vi "Script-Window.vi"(7 "Name(\"\" to use uuid)":string="CSM-Script-Window") -> ()   [LabVIEW 2017, in "DebugConsole.lvlib"]
uses:
  DebugConsole.lvlib
  _BroadcastDef.ctl
  3367f4d9-0615-441f-a9d9-7b84bb446da0.vi
  bf08bd7f-6dab-4e10-8f7c-f5bade8a8a48.vi
  AdvanceAPI/CSM - Revert Arguments-Safe String.vi
  AdvanceAPI/CSM - Keywords.vi
  _csmlite/_PassAllowedMessage - Mapping.vi
  _Shared/Trim Single-line Text.vi
  _Polymophic/Build Synchronous Message with Arguments.vi
  _Polymophic/Build Asynchronous Message with Arguments.vi
  <vilib>/Utility/Data Type/Get Type Information.vi
  _csmHelper/lvcsmFile/lvcsm File Path.vi
  <vilib>/Utility/config.llb/Open Config Data.vi
  <vilib>/Utility/config.llb/Read Key.vi
  <vilib>/Utility/config.llb/Read Key (Boolean).vi
  <vilib>/Utility/config.llb/Read Key (String).vi
  <vilib>/Utility/Data Type/Get Array Information.vi
  <vilib>/Utility/config.llb/Get Key Names.vi
  _csmHelper/lvcsmFile/Path to lvcsm String.vi
  _csmHelper/lvcsmFile/lvcsm String to Path.vi
  <vilib>/Utility/config.llb/Read Key (I32).vi
  <vilib>/Utility/config.llb/Read Key (Double).vi
  <vilib>/Utility/config.llb/Close Config Data.vi
  _csmHelper/lvcsmFile/_Array of VData to VCluster.vi
  <vilib>/Utility/config.llb/Write Key.vi
  <vilib>/Utility/config.llb/Write Key (Boolean).vi
  <vilib>/Utility/config.llb/Remove Key.vi
  <vilib>/Utility/config.llb/Write Key (String).vi
  <vilib>/Utility/config.llb/Write Key (I32).vi
  <vilib>/Utility/config.llb/Write Key (Double).vi
  Communicable State Machine.lvlib
  _csmlite/_csmlite.lvlib
  _csmHelper/lvcsmFile/lvcsm File Support.lvlib
  _Shared/CSM Shared.lvlib
panel:
  in  "List":string(combo)
  in  "Delete":bool
  in  "Save":bool
  out "Running":bool
  in  "Stop":bool
  in  "Play":bool
  in  "Refresh":bool
  in  "Scripts":i32(listbox)
  out "statusbar":string
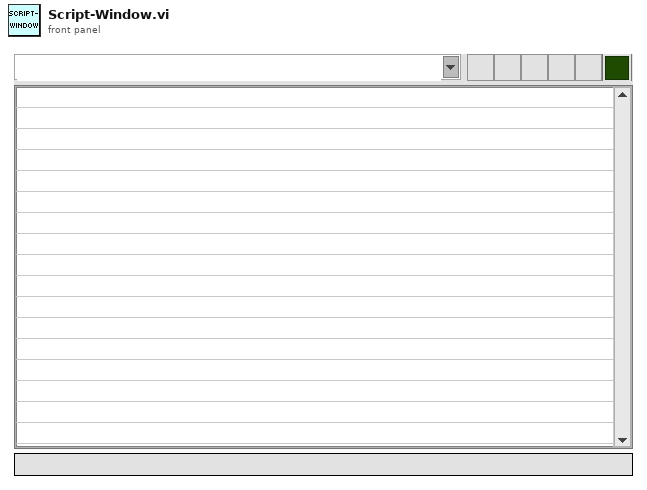
[diagram p1: front panel]
types:
  T1 = enum32{"Invalid", "Standard", "Closed", "Hidden", "Minimized", "Maximized"}
  T2 = enum32{"invalid app kind", "Development System", "Run Time System", "Student Edition", "Embedded LabVIEW", "Evaluation", "Custom"}
  T3 = typedef "DebugConsole.lvlib/_BroadcastDef.ctl" = enum16{"<no action>", "Macro: Exit", "CSM: Module List Changed", "CSM: Scripts Changed", "CSM: Registration Changed", "CSM: Module Selected", "CSM: Message Excuted", "CSM: Broadcast Excuted", "CSM: Registration Action Excuted"}
  T4 = typedef "LVPoint32TypeDef.ctl" = cluster{"Horizontal":i32, "Vertical":i32}
  T5 = cluster{"Current VI Reference":refnum<vi>, "Close Panel on Exit?":bool}
  T6 = cluster{"Core":cluster{"Current VI Reference":refnum<vi>, "Close Panel on Exit?":bool}, "CSMScripts":cluster{"Value":string, "Scripts":cluster{"Target":string, "Function":string, "Parameters":string, "Async Call?":bool}[]}[]}
  T7 = cluster{"Value":string, "Scripts":cluster{"Target":string, "Function":string, "Parameters":string, "Async Call?":bool}[]}[]
  T8 = cluster{"Value":string, "Scripts":cluster{"Target":string, "Function":string, "Parameters":string, "Async Call?":bool}[]}
  T9 = cluster{"Target":string, "Function":string, "Parameters":string, "Async Call?":bool}[]
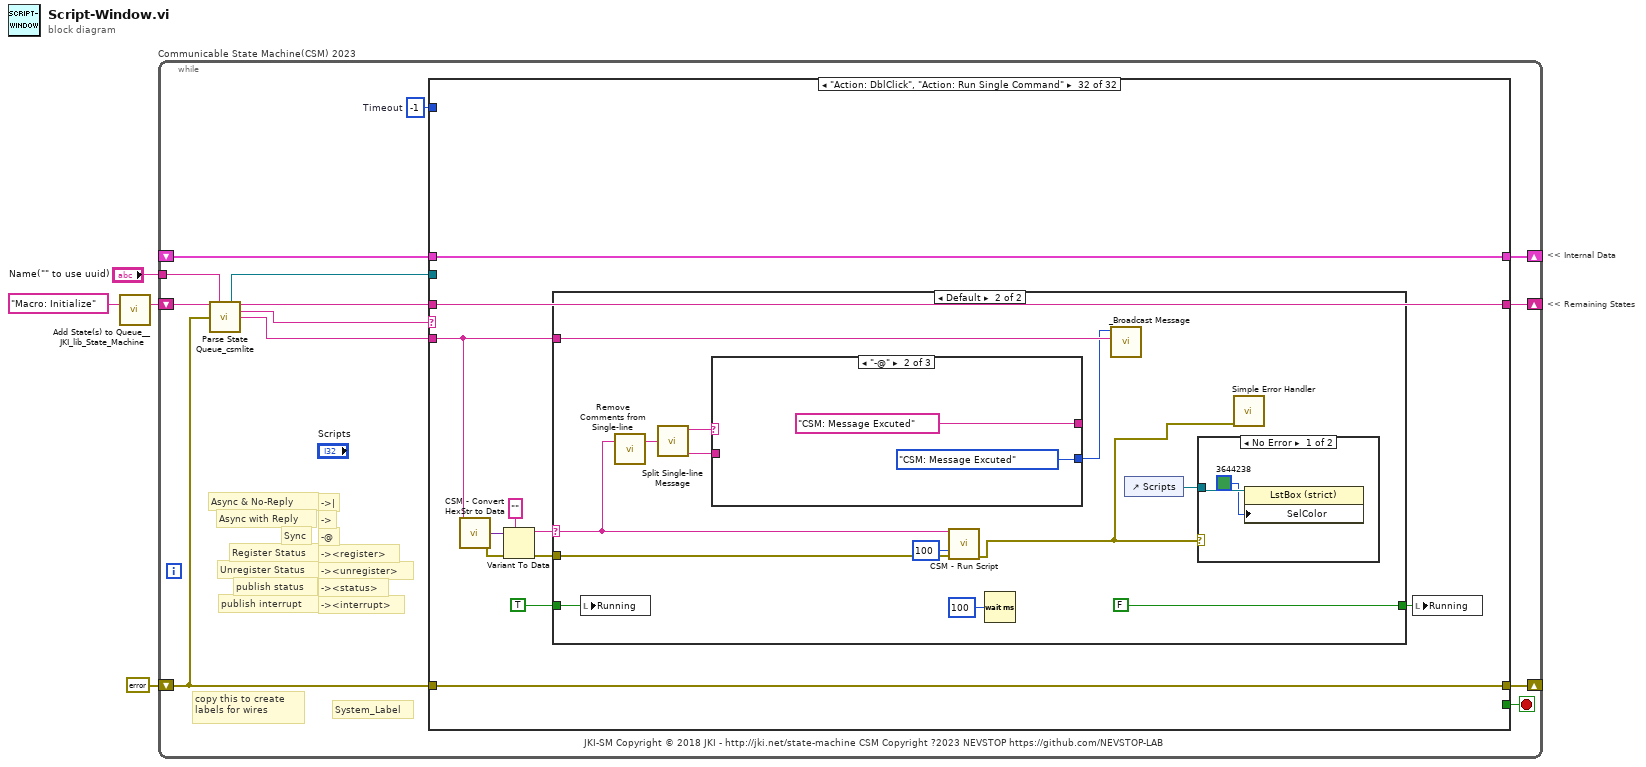
[diagram p0: block diagram]
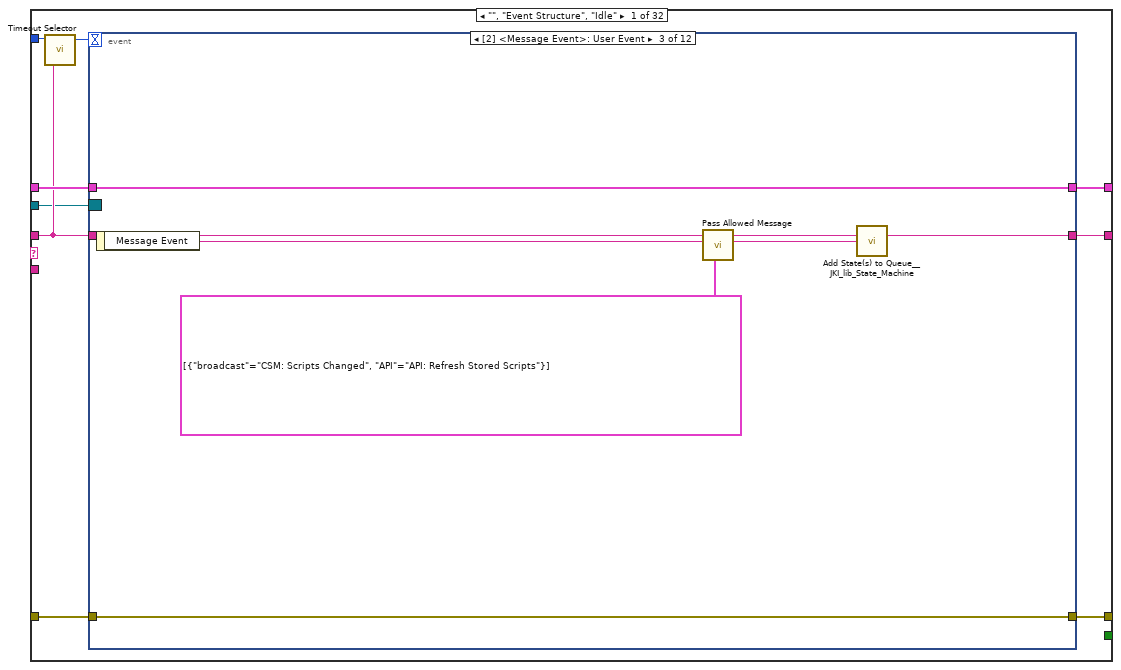
[diagram p2: hidden frame]
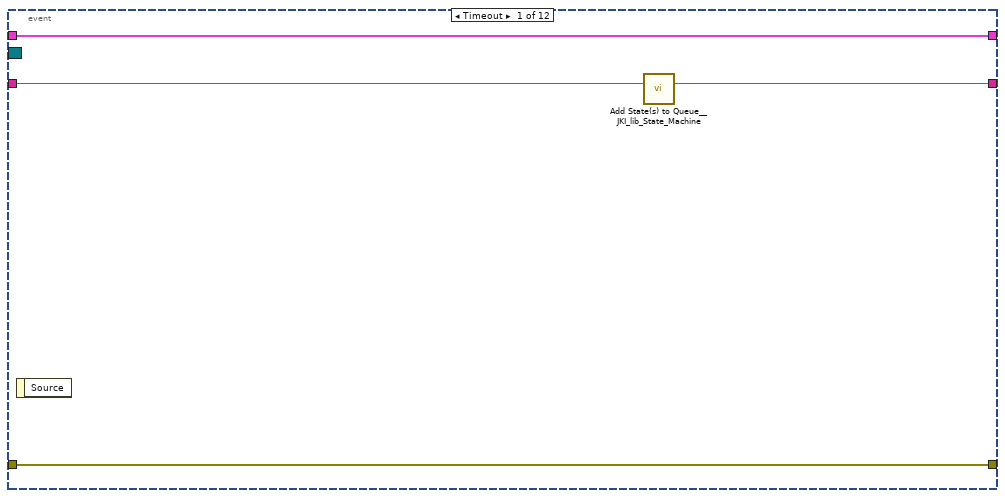
[diagram p3: hidden frame]
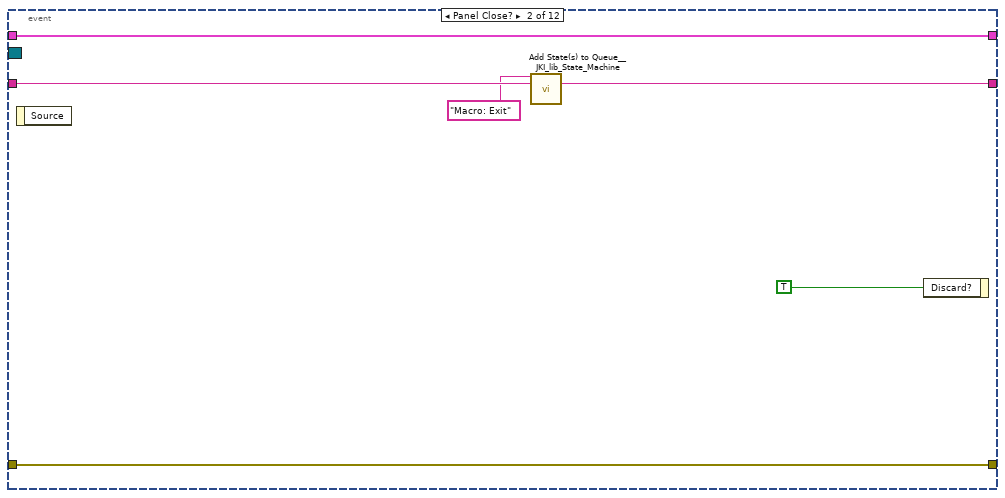
[diagram p4: hidden frame]
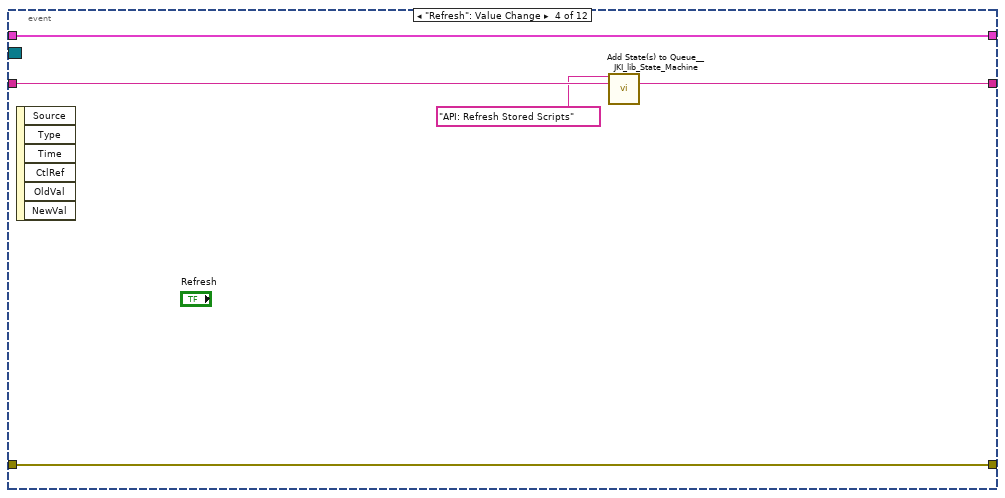
[diagram p5: hidden frame]
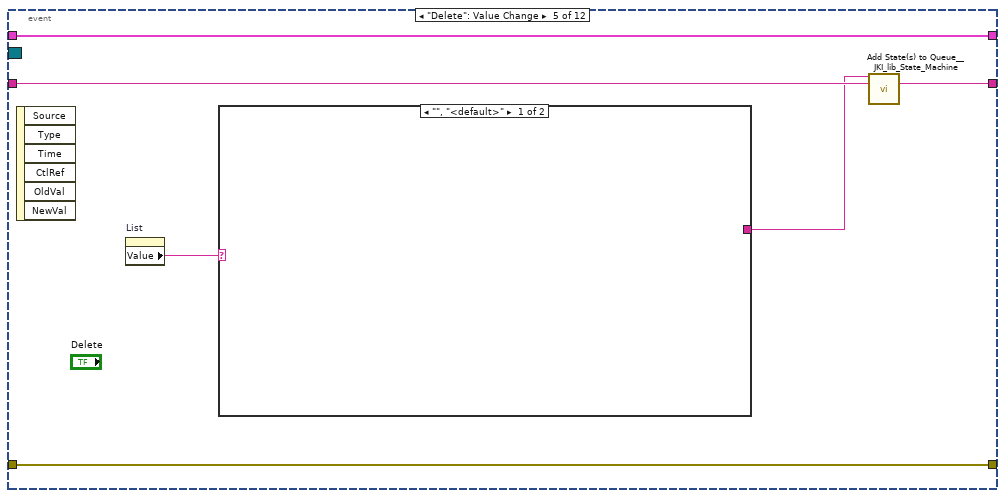
[diagram p6: hidden frame]
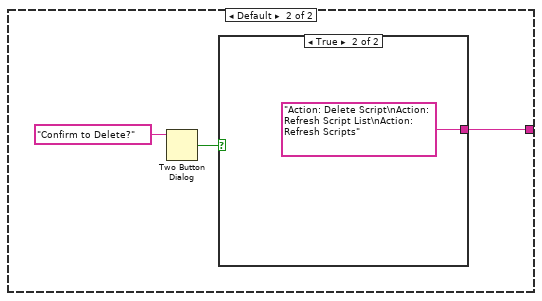
[diagram p7: hidden frame]
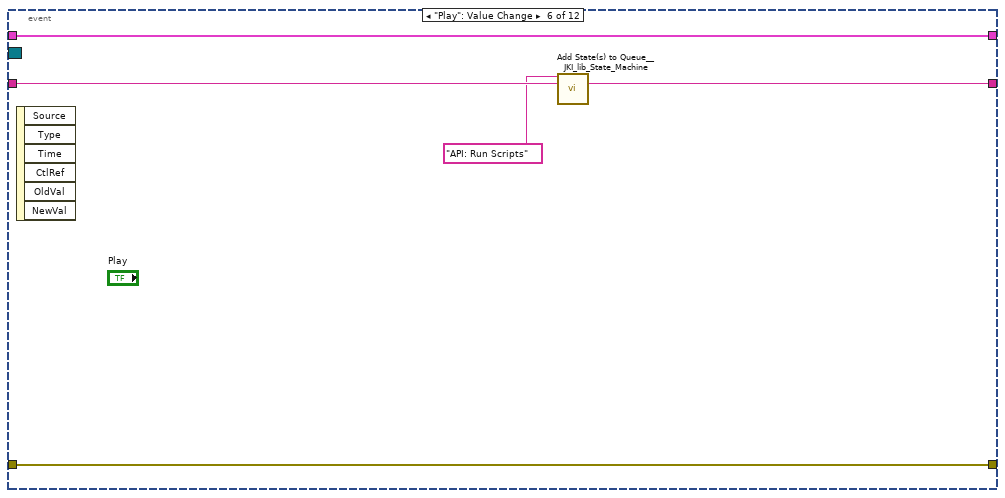
[diagram p9: hidden frame]
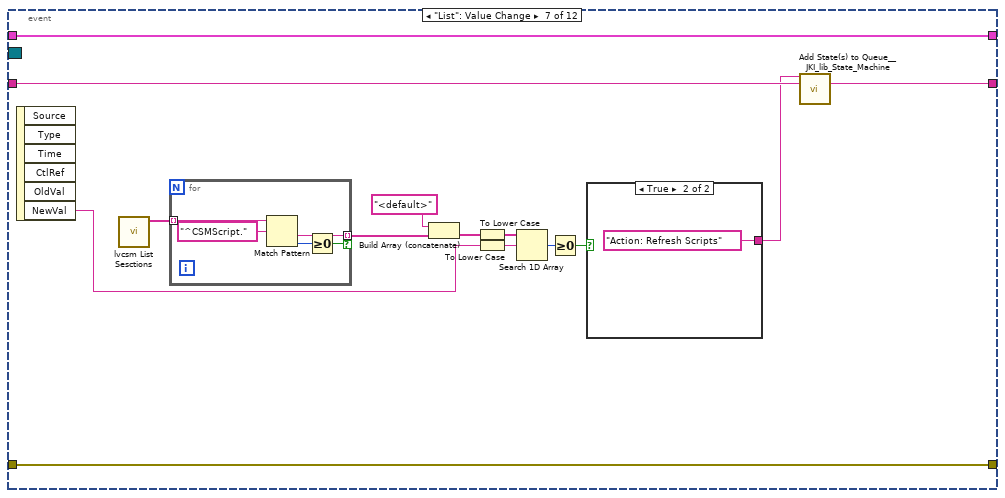
[diagram p10: hidden frame]
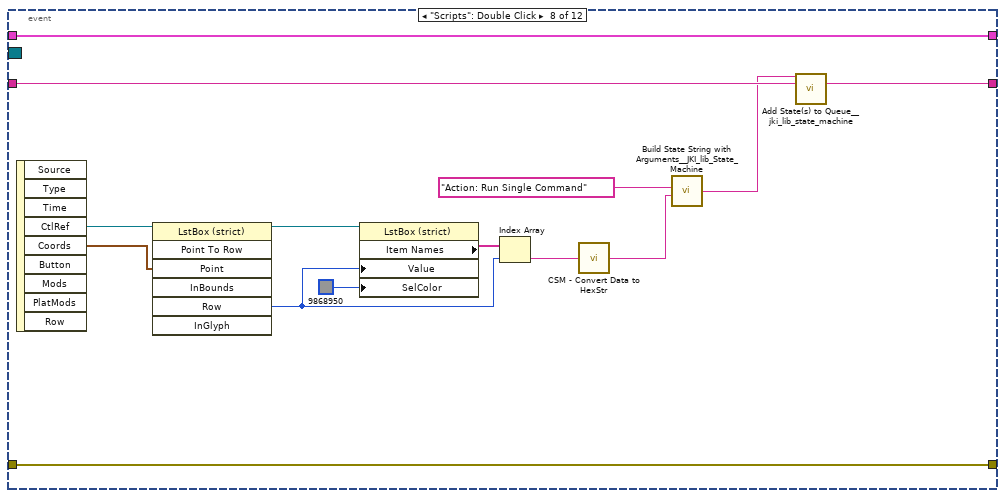
[diagram p12: hidden frame]
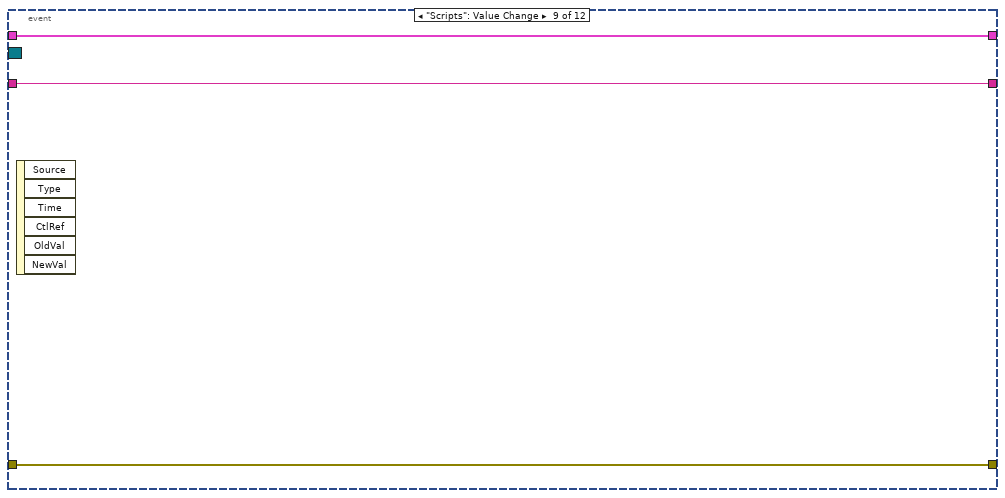
[diagram p13: hidden frame]
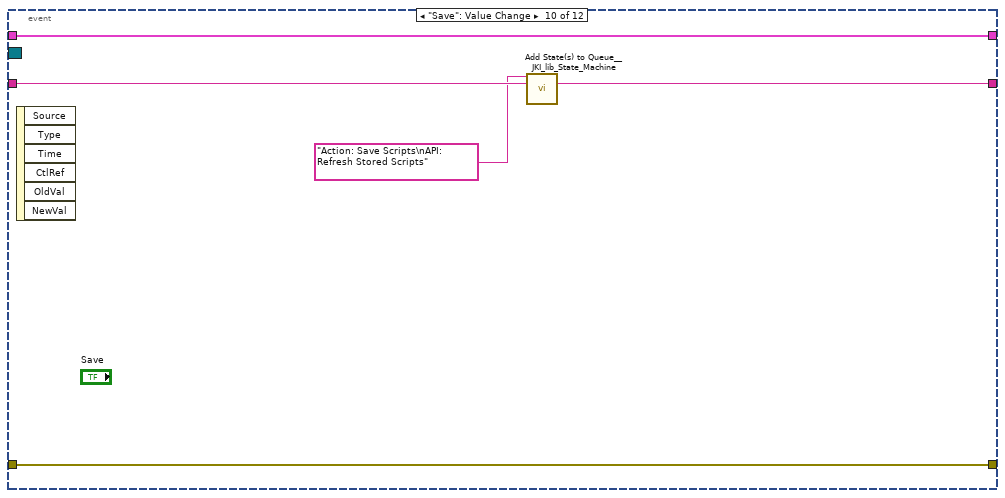
[diagram p14: hidden frame]
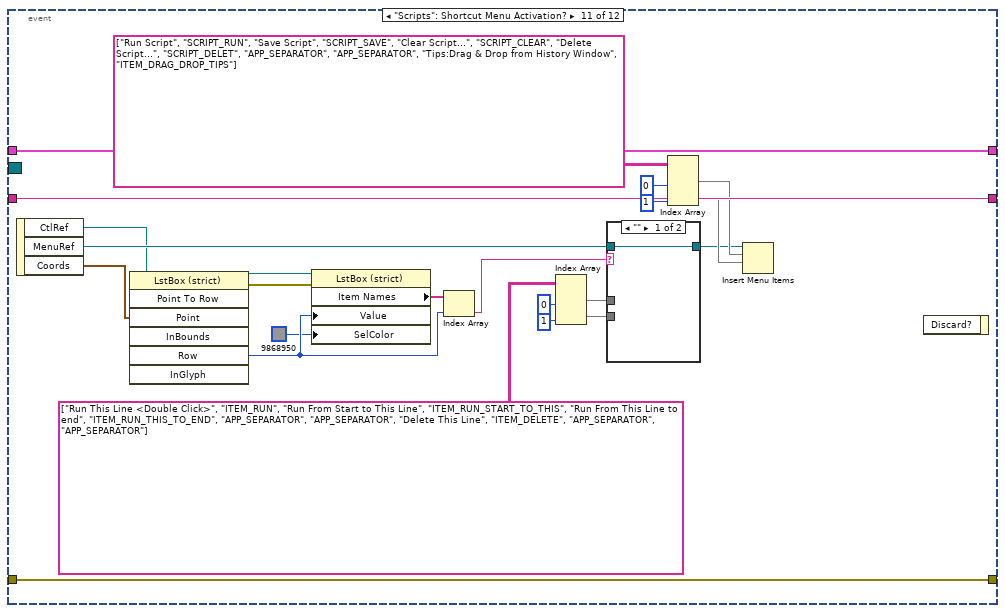
[diagram p15: hidden frame]
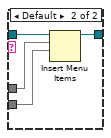
[diagram p16: hidden frame]
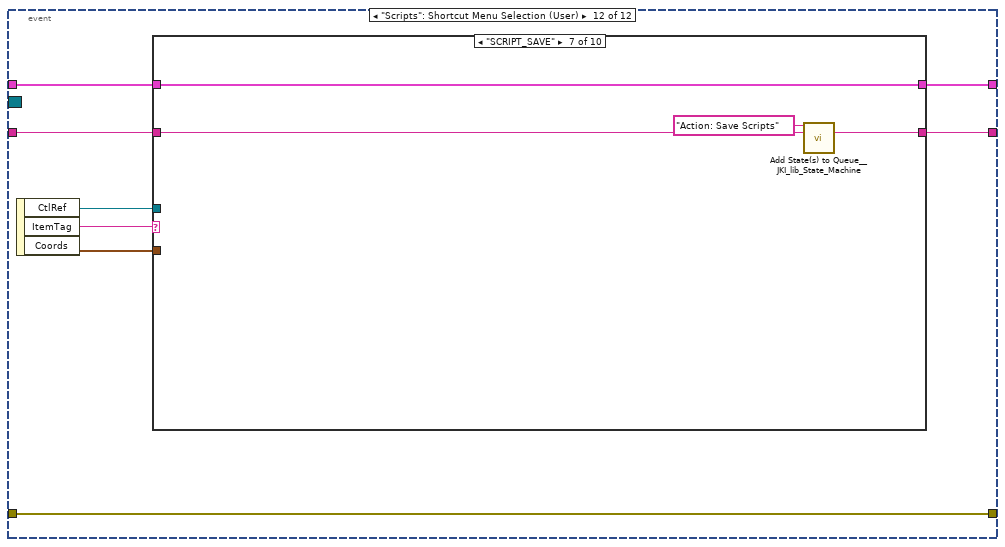
[diagram p17: hidden frame]
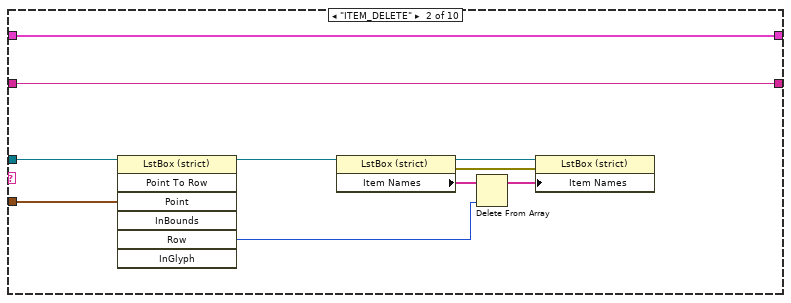
[diagram p19: hidden frame]
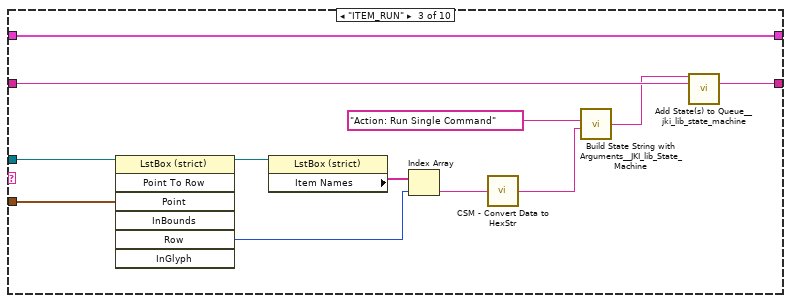
[diagram p20: hidden frame]
diagram:
  # "<< Internal Data"
  # "<< Remaining States"
  n1 = call <vilib>:"Add State(s) to Queue__JKI_lib_State_Machine.vi"("State(s) in (\"\")"="Macro: Initialize" ("Init State(\"Macro: Initialize\")")) -> ("States Out"=w1:string)  [unwired: 14 in]
  n2 = while "Communicable State Machine(CSM) 2023" {
    shift-right: [w12] -> _
    shift-left: _ -> [w11]
    shift-right: [w15] -> _
    shift-left: errorcluster {"status"=FALSE, "code"=0, "source"=""} ("error out") -> [w9]
    shift-right: [w14] -> _
    shift-left: w1 -> [w16]
    tunnel: "Name(\"\" to use uuid)" -> [w8]
    stop <- w13 stop-if-true
    w10 = -1  # Timeout
    # "-><interrupt>"
    # "-><status>"
    # "-><unregister>"
    # "-><register>"
    # "-@"
    # "->"
    # "->|"
    # "publish interrupt"
    # "publish status"
    # "Unregister Status"
    # "Register Status"
    # "Sync"
    # "Async with Reply"
    # "Async & No-Reply"
    # "copy this to create labels for wires"
    # "System_Label"
    # "JKI-SM Copyright © 2018 JKI - http://jki.net/state-machine CSM Copyright ?2023 NEVSTOP https://github.com/NEVSTOP-LAB"
    n3 = call "Parse State Queue_csmlite.vi"("State Queue"=w16, "Current Module(\"\" to generate an ID)"=w8, "Error In (no error)"=w9) -> ("Event Registration Refnum"=w6:refnum<event-registration>, "Remaining States"=w17:string, "Current State"=w7:string, "Arguments"=w5:string)  [unwired: 9 in]
    n4 = case shown="\"Action: DblClick\", \"Action: Run Single Command\"" w7 {
      selector: w7 -> [_ _ _ w206 _ _ _ _ _ _ _ _ _ _ _ _ _ _ _ _ _ _ _ _ _ _ _ _ _ _ _ _]
      tunnel: w17 -> [w19 w201 w205 w210 w219 w234 w250 w255 w259 w265 w271 w275 w279 w284 w293 w311 w333 w348 w417 w422 w433 w435 w451 w496 w540 w571 w576 w591 w606 w608 w624 w637]
      tunnel: w5 -> [_ _ _ _ w217 _ _ _ _ _ _ _ _ _ _ _ w328 w342 _ _ _ _ _ _ _ _ _ _ _ _ _ w632]
      tunnel: w11 -> [w25 w200 w202 w208 w224 w237 w243 w253 w256 _ w266 w272 w276 w282 w292 w310 w331 w344 w414 w419 w430 w434 w448 w493 w537 w573 w575 w590 w605 w612 w623 w636]
      tunnel: [w24 w199 w203 w212 errorcluster {"status"=FALSE, "code"=0, "source"=""} ("error out") w233 w247 w252 w257 w262 w267 w273 w277 w281 _ _ w329 w345 w415 w420 w431 w436 w449 w494 w538 w574 w577 w592 w607 w613 w625 w638] -> w15
      tunnel: w9 -> [w23 w199 w203 w211 w223 w233 w247 w252 w257 w262 w268 w273 w277 w281 _ _ w330 w346 w415 w420 w431 w436 w449 w494 w538 w574 w577 w592 w607 w613 w625 w638]
      tunnel: [w26 w201 w204 w209 w221 w234 w249 w254 w258 w264 w270 w274 w278 w283 w293 w311 w332 w347 w416 w421 w432 w435 w450 w495 w539 w572 w576 w591 w606 w609 w624 w637] -> w14
      tunnel: [_ _ _ _ _ _ _ TRUE _ _ _ _ _ _ _ _ _ _ _ _ _ _ _ _ _ _ _ _ _ _ _ _] -> w13
      tunnel: [w22 w200 w202 w208 w224 w237 w248 w253 w256 w263 w266 w272 w276 w282 w292 w310 w331 w344 w414 w419 w430 w434 w448 w493 w537 w573 w575 w590 w605 w612 w623 w636] -> w12
      tunnel: w10 -> [w21 _ _ _ _ _ _ _ _ _ _ _ _ _ _ _ _ _ _ _ _ _ _ _ _ _ _ _ _ _ _ _]
      tunnel: w6 -> [w18 _ _ _ _ _ _ _ _ _ _ _ _ _ _ _ _ _ _ _ _ _ _ _ _ _ _ _ _ _ _ _]
      frame "", "Event Structure", "Idle" {
        n5 = call "Timeout Selector.vi"("Remaining States"=w19, "Timeout Expected"=w21) -> ("Timeout"=w20:i32)  [unwired: 5 in]
        n6 = event shown="[2] <Message Event>: User Event" {
          selector: w18 -> [_ _ _ _ _ _ _ _ _ _ _ _]
          dyn-events: _ -> [_ _ _ _ _ _ _ _ _ _ _ _]
          timeout: w20 -> [_ _ _ _ _ _ _ _ _ _ _ _]
          tunnel: w19 -> [w30 w36 w40 w45 w51 w60 w74 w94 w100 w102 w128 w137]
          tunnel: [w29 w35 w41 w46 w52 w61 w75 w95 w100 w103 w128 w138] -> w26
          tunnel: w25 -> [w27 w33 w42 w47 w53 w62 w76 w96 w98 w104 w126 w140]
          tunnel: [w28 w34 w43 w48 w54 w63 w77 w97 w99 w105 w127 w141] -> w24
          tunnel: w23 -> [w28 w34 w43 w48 w54 w63 w77 w97 w99 w105 w127 w141]
          tunnel: [w27 w33 w42 w47 w53 w62 w76 w96 w98 w104 w126 w139] -> w22
          event Timeout {
            n7 = event-data() -> ()  [unwired: 1 in, 1 out]
            n8 = call <vilib>:"Add State(s) to Queue__JKI_lib_State_Machine.vi"("State(s) in (\"\")"=w30) -> ("States Out"=w29:string)  [unwired: 14 in]
          }
          event Panel Close? {
            n9 = event-data() -> ()  [unwired: 1 in, 1 out]
            n10 = call <vilib>:"Add State(s) to Queue__JKI_lib_State_Machine.vi"("State(s) in Front (\"\")"="Macro: Exit", "State(s) in (\"\")"=w36) -> ("States Out"=w35:string)  [unwired: 13 in]
            n11 = event-data("Discard?"=TRUE) -> ()  [unwired: 1 in, 1 out]
          }
          event User Event {
            n12 = event-data() -> ("Message Event"=w39:string)  [unwired: 1 in]
            n13 = call-poly "Pass Allowed Message.vi"("Mapping"=cluster{"broadcast":string, "API":string}[] [{"broadcast"="CSM: Scripts Changed", "API"="API: Refresh Stored Scripts"}], "JKISM External Event"=w39) -> ("States"=w38:string)  [unwired: 7 in]
            n14 = call <vilib>:"Add State(s) to Queue__JKI_lib_State_Machine.vi"("State(s) in (\"\")"=w40, "State(s) at Back (\"\")"=w38) -> ("States Out"=w41:string)  [unwired: 13 in]
          }
          event "Refresh": Value Change {
            n15 = event-data() -> ()  [unwired: 1 in, 6 out]
            n16 = call <vilib>:"Add State(s) to Queue__JKI_lib_State_Machine.vi"("State(s) in Front (\"\")"="API: Refresh Stored Scripts" ("State(s) in Front (\"\")"), "State(s) in (\"\")"=w45) -> ("States Out"=w46:string)  [unwired: 13 in]
          }
          event "Delete": Value Change {
            n17 = event-data() -> ()  [unwired: 1 in, 6 out]
            n18 = property on="List" class="CmbBox"() -> ("Value"=w49:string)  [unwired: 2 in, 2 out]
            n19 = case shown="\"\", \"<default>\"" w49 {
              tunnel: [_ w57] -> w50
              frame "", "<default>" {
              }
              frame Default {
                n20 = Two Button Dialog(message="Confirm to Delete?") -> (T button?=w55:bool)  [unwired: 2 in]
                n21 = case shown="True" w55 {
                  tunnel: [_ "Action: Delete Script\nAction: Refresh Script List\nAction: Refresh Scripts" ("State(s) in Front (\"\")")] -> w57
                  frame False {
                  }
                  frame True {
                  }
                }
              }
            }
            n22 = call <vilib>:"Add State(s) to Queue__JKI_lib_State_Machine.vi"("State(s) in Front (\"\")"=w50, "State(s) in (\"\")"=w51) -> ("States Out"=w52:string)  [unwired: 13 in]
          }
          event "Play": Value Change {
            n23 = event-data() -> ()  [unwired: 1 in, 6 out]
            n24 = call <vilib>:"Add State(s) to Queue__JKI_lib_State_Machine.vi"("State(s) in Front (\"\")"="API: Run Scripts" ("State(s) in Front (\"\")"), "State(s) in (\"\")"=w60) -> ("States Out"=w61:string)  [unwired: 13 in]
          }
          event "List": Value Change {
            n25 = event-data() -> ("NewVal"=w71:string)  [unwired: 1 in, 5 out]
            n26 = call "lvcsm List Sesctions.vi"() -> ("Section Names"=w72:string[])  [unwired: 10 in, 1 out]
            n27 = for {
              tunnel: w72 -> [w83] mode=indexing
              tunnel: [w81] -> w65 mode=indexing if=w79
              n28 = Match Pattern(string=w83, regular expression="^CSMScript.") -> (after substring=w81:string, offset past match=w80:i32)  [unwired: 1 in, 2 out]
              n29 = Greater Or Equal To 0?(x=w80) -> (x >= 0?=w79:bool)
            }
            n30 = Build Array (concatenate)("<default>" ("regular expression"), w65) -> (w64:string[])
            n31 = To Lower Case(string=w64) -> (all lower case string=w69:string[])
            n32 = To Lower Case(string=w71) -> (all lower case string=w70:string)
            n33 = Search 1D Array(1D array=w69, element=w70) -> (index of element=w68:i32)  [unwired: 1 in]
            n34 = Greater Or Equal To 0?(x=w68) -> (x >= 0?=w67:bool)
            n35 = case shown="True" w67 {
              tunnel: [_ "Action: Refresh Scripts" ("State(s) in Front (\"\")")] -> w73
              frame False {
              }
              frame True {
              }
            }
            n36 = call <vilib>:"Add State(s) to Queue__JKI_lib_State_Machine.vi"("State(s) in Front (\"\")"=w73, "State(s) in (\"\")"=w74) -> ("States Out"=w75:string)  [unwired: 13 in]
          }
          event "Scripts": Double Click {
            n37 = event-data() -> ("CtlRef"=w88:refnum<vi>, "Coords"=w87:T4)  [unwired: 1 in, 7 out]
            n38 = invoke class="LstBox (strict)" method="Point To Row"(reference=w88, "Point"=w87) -> (reference out=w92:refnum<vi>, "Row"=w85:i32)  [unwired: 5 in, 5 out]
            n39 = property class="LstBox (strict)"(reference=w92, "Value"=w85, "SelColor"=u32 9868950) -> ("Item Names"=w93:string[])  [unwired: 1 in, 2 out]
            n40 = Index Array(array=w93, index=w85) -> (element=w91:string)
            n41 = call "CSM - Convert Data to HexStr.vi"("Variant"=w91) -> ("HEX String (0-9,A-F)"=w90:string)  [unwired: 8 in]
            n42 = call <vilib>:"Build State String with Arguments__JKI_lib_State_Machine.vi"("Arguments (\"\")"=w90, "State"="Action: Run Single Command" ("State(s) in Front (\"\")")) -> ("State with Arguments"=w86:string)  [unwired: 4 in]
            n43 = call <vilib>:"Add State(s) to Queue__jki_lib_state_machine.vi"("State(s) in Front (\"\")"=w86, "State(s) in (\"\")"=w94) -> ("States Out"=w95:string)  [unwired: 13 in]
          }
          event "Scripts": Value Change {
            n44 = event-data() -> ()  [unwired: 1 in, 6 out]
          }
          event "Save": Value Change {
            n45 = event-data() -> ()  [unwired: 1 in, 6 out]
            n46 = call <vilib>:"Add State(s) to Queue__JKI_lib_State_Machine.vi"("State(s) in Front (\"\")"="Action: Save Scripts\nAPI: Refresh Stored Scripts" ("State(s) in Front (\"\")"), "State(s) in (\"\")"=w102) -> ("States Out"=w103:string)  [unwired: 13 in]
          }
          event "Scripts": Shortcut Menu Activation? {
            n47 = event-data() -> ("CtlRef"=w109:refnum<vi>, "MenuRef"=w112:refnum<k9>, "Coords"=w108:T4)  [unwired: 1 in]
            n48 = invoke class="LstBox (strict)" method="Point To Row"(reference=w109, "Point"=w108) -> (reference out=w111:refnum<vi>, error out=w110:errorcluster, "Row"=w107:i32)  [unwired: 5 in, 4 out]
            n49 = property class="LstBox (strict)"(reference=w111, error in=w110, "Value"=w107, "SelColor"=u32 9868950) -> ("Item Names"=w120:string[])  [unwired: 2 out]
            n50 = Index Array(array=w120, index=w107) -> (element=w113:string)
            n51 = Index Array(array=string[][] [["Run This Line <Double Click>", "ITEM_RUN"], ["Run From Start to This Line", "ITEM_RUN_START_TO_THIS"], ["Run From This Line to end", "ITEM_RUN_THIS_TO_END"], ["APP_SEPARATOR", "APP_SEPARATOR"], ["Delete This Line", "ITEM_DELETE"], ["APP_SEPARATOR", "APP_SEPARATOR"]] ("item names"), index (col) #1=0 ("index (row)"), index (col) #2=1 ("index (row)")) -> (element #1=w116:string[], element #2=w114:string[])  [unwired: 2 in]
            n52 = case shown="\"\"" w113 {
              tunnel: [w129 w133] -> w119
              tunnel: w112 -> [w129 w132]
              tunnel: w116 -> [_ w131]
              tunnel: w114 -> [_ w130]
              frame "" {
              }
              frame Default {
                n53 = Insert Menu Items(7:w130, 8:w131, 9:w132) -> (3:w133:refnum<k9>)  [unwired: 3 in, 2 out]
              }
            }
            n54 = Index Array(array=string[][] [["Run Script", "SCRIPT_RUN"], ["Save Script", "SCRIPT_SAVE"], ["Clear Script...", "SCRIPT_CLEAR"], ["Delete Script...", "SCRIPT_DELET"], ["APP_SEPARATOR", "APP_SEPARATOR"], ["Tips:Drag & Drop from History Window", "ITEM_DRAG_DROP_TIPS"]] ("item names"), index (col) #1=0 ("index (row)"), index (col) #2=1 ("index (row)")) -> (element #1=w124:string[], element #2=w123:string[])  [unwired: 2 in]
            n55 = Insert Menu Items(7:w123, 8:w124, 9:w119) -> ()  [unwired: 3 in, 3 out]
            n56 = event-data() -> ()  [unwired: 2 in, 1 out]
          }
          event "Scripts": Shortcut Menu Selection (User) {
            n57 = event-data() -> ("CtlRef"=w135:refnum<vi>, "ItemTag"=w136:string, "Coords"=w134:T4)  [unwired: 1 in]
            n58 = case shown="\"SCRIPT_SAVE\"" w136 {
              tunnel: w140 -> [w143 w153 w165 w167 w171 w175 w179 w183 w189 w197]
              tunnel: [w142 w152 w164 w166 w170 w174 w178 w182 w188 w196] -> w138
              tunnel: [w143 w153 w165 w167 w171 w175 w179 w183 w189 w197] -> w139
              tunnel: w137 -> [w142 w152 w163 w166 w169 w173 w177 w181 w187 w195]
              tunnel: w135 -> [_ w151 w156 _ _ _ _ _ _ _]
              tunnel: w134 -> [_ w145 w155 _ _ _ _ _ _ _]
              frame Default {
              }
              frame "ITEM_DELETE" {
                n59 = invoke class="LstBox (strict)" method="Point To Row"(reference=w151, "Point"=w145) -> (reference out=w146:refnum<vi>, "Row"=w144:i32)  [unwired: 5 in, 5 out]
                n60 = property class="LstBox (strict)"(reference=w146) -> (reference out=w150:refnum<vi>, error out=w149:errorcluster, "Item Names"=w148:string[])  [unwired: 1 in]
                n61 = Delete From Array(array=w148, index=w144) -> (array with subset deleted=w147:string[])  [unwired: 1 in, 1 out]
                n62 = property class="LstBox (strict)"(reference=w150, error in=w149, "Item Names"=w147) -> ()  [unwired: 2 out]
              }
              frame "ITEM_RUN" {
                n63 = invoke class="LstBox (strict)" method="Point To Row"(reference=w156, "Point"=w155) -> (reference out=w161:refnum<vi>, "Row"=w160:i32)  [unwired: 5 in, 5 out]
                n64 = property class="LstBox (strict)"(reference=w161) -> ("Item Names"=w162:string[])  [unwired: 1 in, 2 out]
                n65 = Index Array(array=w162, index=w160) -> (element=w157:string)
                n66 = call "CSM - Convert Data to HexStr.vi"("Variant"=w157) -> ("HEX String (0-9,A-F)"=w154:string)  [unwired: 8 in]
                n67 = call <vilib>:"Build State String with Arguments__JKI_lib_State_Machine.vi"("Arguments (\"\")"=w154, "State"="Action: Run Single Command" ("State(s) in Front (\"\")")) -> ("State with Arguments"=w158:string)  [unwired: 4 in]
                n68 = call <vilib>:"Add State(s) to Queue__jki_lib_state_machine.vi"("State(s) in Front (\"\")"=w158, "State(s) in (\"\")"=w163) -> ("States Out"=w164:string)  [unwired: 13 in]
              }
              frame "ITEM_DRAG_DROP_TIPS" {
              }
              frame "SCRIPT_RUN" {
                n69 = call <vilib>:"Add State(s) to Queue__JKI_lib_State_Machine.vi"("State(s) in Front (\"\")"="API: Run Scripts" ("State(s) in Front (\"\")"), "State(s) in (\"\")"=w169) -> ("States Out"=w170:string)  [unwired: 13 in]
              }
              frame "ITEM_RUN_START_TO_THIS" {
                n70 = call <vilib>:"Add State(s) to Queue__JKI_lib_State_Machine.vi"("State(s) in Front (\"\")"="API: Run Scripts From Start to This Line" ("State(s) in Front (\"\")"), "State(s) in (\"\")"=w173) -> ("States Out"=w174:string)  [unwired: 13 in]
              }
              frame "SCRIPT_SAVE" {
                n71 = call <vilib>:"Add State(s) to Queue__JKI_lib_State_Machine.vi"("State(s) in Front (\"\")"="Action: Save Scripts" ("State(s) in Front (\"\")"), "State(s) in (\"\")"=w177) -> ("States Out"=w178:string)  [unwired: 13 in]
              }
              frame "ITEM_RUN_THIS_TO_END" {
                n72 = call <vilib>:"Add State(s) to Queue__JKI_lib_State_Machine.vi"("State(s) in Front (\"\")"="API: Run Scripts From This Line to End" ("State(s) in Front (\"\")"), "State(s) in (\"\")"=w181) -> ("States Out"=w182:string)  [unwired: 13 in]
              }
              frame "SCRIPT_CLEAR" {
                n73 = Two Button Dialog(message="Confirm to clear all?") -> (T button?=w185:bool)  [unwired: 2 in]
                n74 = case shown="True" w185 {
                  tunnel: [_ "Action: Save Scripts\nAPI: Refresh Stored Scripts" ("State(s) in Front (\"\")")] -> w186
                  frame False {
                  }
                  frame True {
                    n75 = property on="Scripts" class="LstBox (strict)"("Item Names"=string[] []) -> ()  [unwired: 2 in, 2 out]
                  }
                }
                n76 = call <vilib>:"Add State(s) to Queue__JKI_lib_State_Machine.vi"("State(s) in Front (\"\")"=w186, "State(s) in (\"\")"=w187) -> ("States Out"=w188:string)  [unwired: 13 in]
              }
              frame "SCRIPT_DELET" {
                n77 = Two Button Dialog(message="Confirm to delete?") -> (T button?=w193:bool)  [unwired: 2 in]
                n78 = case shown="True" w193 {
                  tunnel: [_ "Action: Delete Script\nAPI: Refresh Stored Scripts" ("State(s) in Front (\"\")")] -> w194
                  frame False {
                  }
                  frame True {
                  }
                }
                n79 = call <vilib>:"Add State(s) to Queue__JKI_lib_State_Machine.vi"("State(s) in Front (\"\")"=w194, "State(s) in (\"\")"=w195) -> ("States Out"=w196:string)  [unwired: 13 in]
              }
            }
          }
        }
      }
      frame "CSM Documentation" {
      }
      frame "---------- Core ----------" {
        n80 = call <vilib>:"Add State(s) to Queue__JKI_lib_State_Machine.vi"("State(s) in (\"\")"=w205) -> ("States Out"=w204:string)  [unwired: 14 in]
      }
      frame Default {
        w215 = 42 items=["No error", "Argument error", "Memory is full", "Out of zone", "End of file", "File already open", "Generic file I/O error", "File not found", "File permission error", "Disk is full", "Duplicate path", "Too many files open", "System feature not enabled", "Resource file not found", "Cannot add resource", "Resource not found", "Image not found", "Image memory error", "Pen does not exist", "Config type invalid", "Config token not found", "Config parse error", "Config memory error", "Bad external code format", "Bad external code offset", "External code not present", "Null window", "Destroy window error", "Null menu", "Print aborted", "Bad print record", "Print driver error", "Windows error during printing", "Memory error during printing", "Print dialog error", "Generic print error", "Invalid device refnum", "Device not found", "Device parameter error", "Device unit error", "Cannot open device", "Device call aborted", "Generic error", "Cancelled by user", "Object ID too low", "Object ID too high", "Object not in heap", "Unknown heap", "Unknown object (invalid DefProc)", "Unknown object (DefProc not in table)", "Message out of range", "Invalid (null) method", "Unknown message", "Manager call not supported", "Bad address", "Network operation in progress", "Network operation timed out", "Connection is busy", "Network attribute not supported", "Network error", "Address in use", "System out of memory", "Connection aborted", "Connection refused", "Not connected", "Already connected", "Connection closed", "Initialization error (interapplication manager)", "Bad occurrence", "Wait on unbound occurrence handler", "Occurrence queue overflow", "Datalog type conflict", "Unused", "Unrecognized type (interapplication manager)", "Memory corrupt", "Failed to make temporary DLL", "Old CIN version", "Drag socket not found", "Failed to load drop-object", "Failed to register OLE object", "Failed to release OLE object", "Format specifier type mismatch", "Unknown format specifier", "Too few format specifiers", "Too many format specifiers", "Scan failed", "Newer CIN version", "Error converting to variant", "Runtime menu error", "Password tampered", "Variant attribute not found", "Incompatible variant data type", "Event data is not available", "Event Store is not present", "Occurrence is not found", "Event Queue is not created", "Event info is not available", "Refnum passed is NULL", "Error retrieving Class GUID", "Error retrieving CoClass GUID", "Error retrieving TypeLib GUID.", "Bad built application magic bytes.", "Specific driver is different from the specific driver associated with the Logical Name.", "There is no session opened to the class driver.", "Max Error", "MAX - Error with config objects", "MAX - Error loading configuration", "MAX - Group not supported"]
        # "Handle mistyped state name (developer tool)"
        n81 = Format Into String(format string="Software Exception: Unhandled State \"%s\"." ("message"), error in=w211, w206) -> (resulting string=w214:string, error out=w213:errorcluster)  [unwired: 1 in]
        n82 = call <vilib>:"Error Cluster From Error Code.vi"("show call chain? (False)"=TRUE, "error in (no error)"=w213, "error message (\"\")"=w214, "error code (0)"=w215) -> ("error out"=w212:errorcluster)  [unwired: 5 in]
        n83 = call <vilib>:"Add State(s) to Queue__JKI_lib_State_Machine.vi"("State(s) in (\"\")"=w210) -> ("States Out"=w209:string)  [unwired: 14 in]
      }
      frame "Error Handler" {
        # "Clear error"
        n84 = case shown="Error" w223 {
          selector: w223 -> [_ w231]
          tunnel: [w229 w232] -> w220
          tunnel: w219 -> [w229 w232]
          tunnel: [w228 w231] -> w218
          tunnel: w217 -> [w230 _]
          frame No Error {
            n85 = call "CSM - Convert Argument to Error.vi"("Argument"=w230) -> ("Error"=w228:errorcluster)  [unwired: 4 in]
            n86 = flat-sequence {
              frame #0 {
              }
            }
          }
          frame Error {
          }
        }
        n87 = disable-structure shown="Enabled" {
          disable-tunnel: w218 -> [w226 w227]
          frame Enabled {
            # "Unhandled Error -- Display it"
            n88 = call <vilib>:"General Error Handler.vi"("error in (no error)"=w226) -> ()  [unwired: 10 in, 5 out]
          }
          frame Disabled {
            n89 = call <vilib>:"Clear Errors.vi"("error in (no error)"=w227) -> ()  [unwired: 5 in, 2 out]
          }
        }
        n90 = call <vilib>:"Add State(s) to Queue__JKI_lib_State_Machine.vi"("State(s) in Front (\"\")"="// Post Error States", "State(s) in (\"\")"=w220) -> ("States Out"=w221:string)  [unwired: 13 in]
      }
      frame "VI Reference" {
        n91 = Unbundle By Name(w237) -> ("Core"=w236:T5)
        n92 = Unbundle By Name(w236) -> ("Current VI Reference"=w235:refnum<vi>)
        n93 = call "CSM - Convert Data to HexStr.vi"("Variant"=w235) -> ()  [unwired: 8 in, 1 out]
      }
      frame "Initialize Core Data" {
        # "originally closed?"
        # "exe?"
        # "If panel starts closed or is an EXE, then close it when we exit"
        n94 = property class="VI"() -> ("FP.State"=w240:T1)  [unwired: 2 in, 2 out]
        n95 = property class="App"() -> ("App.Kind"=w246:T2)  [unwired: 2 in, 2 out]
        n96 = control-ref of="Current VI Reference"() -> (w241:refnum<vi>)
        n97 = Equal?(x=w240, y=T1."Closed" ("Front Panel Window:State")) -> (x = y?=w238:bool)
        n98 = Equal?(x=w246, y=T2."Run Time System" ("Application:Kind")) -> (x = y?=w244:bool)
        n99 = Or(x=w238, y=w244) -> (x .or. y?=w242:bool)
        n100 = Bundle By Name(cluster=w243, "Core.Current VI Reference"=w241, "Core.Close Panel on Exit?"=w242) -> (w248:T6)
        n101 = call <vilib>:"Add State(s) to Queue__JKI_lib_State_Machine.vi"("State(s) in (\"\")"=w250) -> ("States Out"=w249:string)  [unwired: 14 in]
      }
      frame "Exit" {
        n102 = call <vilib>:"Add State(s) to Queue__JKI_lib_State_Machine.vi"("State(s) in (\"\")"=w255) -> ("States Out"=w254:string)  [unwired: 14 in]
      }
      frame "---------- Data ----------" {
        n103 = call <vilib>:"Add State(s) to Queue__JKI_lib_State_Machine.vi"("State(s) in (\"\")"=w259) -> ("States Out"=w258:string)  [unwired: 14 in]
      }
      frame "Data: Initialize" {
        w260 = T7 []  # CSMScripts
        w261 = T5 {"Current VI Reference"=refnum, "Close Panel on Exit?"=FALSE}  # Core
        n104 = Bundle("Core"=w261, "CSMScripts"=w260) -> (w263:T6)  [unwired: 1 in]
        n105 = call <vilib>:"Add State(s) to Queue__JKI_lib_State_Machine.vi"("State(s) in (\"\")"=w265) -> ("States Out"=w264:string)  [unwired: 14 in]
      }
      frame "Data: Cleanup" {
        n106 = Unbundle By Name(w266) -> ("Core.Current VI Reference"=w269:refnum<vi>)
        n107 = Close Reference(reference=w269, error in (no error)=w268) -> (error out=w267:errorcluster)
        n108 = call <vilib>:"Add State(s) to Queue__JKI_lib_State_Machine.vi"("State(s) in (\"\")"=w271) -> ("States Out"=w270:string)  [unwired: 14 in]
      }
      frame "---------- Events ----------" {
        n109 = call <vilib>:"Add State(s) to Queue__JKI_lib_State_Machine.vi"("State(s) in (\"\")"=w275) -> ("States Out"=w274:string)  [unwired: 14 in]
      }
      frame "---------- UI ----------" {
        n110 = call <vilib>:"Add State(s) to Queue__JKI_lib_State_Machine.vi"("State(s) in (\"\")"=w279) -> ("States Out"=w278:string)  [unwired: 14 in]
      }
      frame "UI: Initialize" {
        n111 = call <vilib>:"Add State(s) to Queue__JKI_lib_State_Machine.vi"("State(s) in (\"\")"=w284) -> ("States Out"=w283:string)  [unwired: 14 in]
        "statusbar" <- "Tips: 1. <double Click> to excute selected command.    2. You can edit the script in this window" ("statusbar")
      }
      frame "UI: Refresh CSM Scripts" {
        n112 = Unbundle By Name(w292) -> ("CSMScripts"=w290:T7)
        n113 = for {
          tunnel: w290 -> [w298] mode=indexing
          tunnel: [w297] -> w285 mode=indexing
          n114 = Unbundle By Name(w298) -> ("Value"=w297:string)  [unwired: 1 out]
        }
        n115 = property on="List" class="CmbBox"() -> (error out=w289:errorcluster, "Value"=w286:string)  [unwired: 2 in, 1 out]
        n116 = Empty String/Path?(string/path=w286) -> (empty?=w288:bool)
        n117 = case shown="True" w288 {
          tunnel: [w294 w295] -> w287
          tunnel: w286 -> [w294 _]
          tunnel: w285 -> [_ w296]
          frame False {
          }
          frame True {
            n118 = Index Array(array=w296) -> (element=w295:string)  [unwired: 1 in]
          }
        }
        n119 = property on="List" class="CmbBox"(error in=w289, "Strings[]"=w285, "AllowUndefStrs"=FALSE ("Allow Undefined Strings"), "Value"=w287) -> ()  [unwired: 1 in, 2 out]
      }
      frame "UI: Switch Script" {
        n120 = Unbundle By Name(w310) -> ("CSMScripts"=w309:T7)
        n121 = for {
          tunnel: w309 -> [w327] mode=indexing
          tunnel: [w326] -> w304 mode=indexing
          n122 = Unbundle By Name(w327) -> ("Value"=w326:string)  [unwired: 1 out]
        }
        n123 = Search 1D Array(1D array=w304, element="List") -> (index of element=w302:i32)  [unwired: 1 in]
        n124 = Index Array(array=w309, index=w302) -> (element=w308:T8)
        n125 = Unbundle By Name(w308) -> ("Scripts"=w307:T9)
        n126 = for {
          tunnel: w307 -> [w317] mode=indexing
          tunnel: [w312] -> w306 mode=indexing
          n127 = Unbundle By Name(w317) -> ("Target"=w315:string, "Function"=w314:string, "Parameters"=w313:string, "Async Call?"=w316:bool)
          n128 = case shown="False" w316 {
            tunnel: w315 -> [w318 w323]
            tunnel: w314 -> [w320 w325]
            tunnel: w313 -> [w319 w324]
            tunnel: [w321 w322] -> w312
            frame False {
              n129 = call-poly "Build Message with Arguments++.vi"("State With Arguments"=w320, "Arguments (\"\")"=w319, "Target Module (\"\")"=w318) -> ("CSM Message String"=w321:string)  [unwired: 12 in]
            }
            frame True {
              n130 = call-poly "Build Message with Arguments++.vi"("State With Arguments"=w325, "Arguments (\"\")"=w324, "Target Module (\"\")"=w323) -> ("CSM Message String"=w322:string)  [unwired: 12 in]
            }
          }
        }
        n131 = property on="Scripts" class="LstBox (strict)"("Item Names"=w306, "Value"=-1 ("Scripts"), "SelColor"=u32 3644238, "Top Row"=0) -> ()  [unwired: 2 in, 2 out]
        "Running" <- FALSE ("Running")
      }
      frame "UI: Cursor Set" {
        # "Argument"
        n132 = disable-structure shown="Default" {
          disable-tunnel: w330 -> [w336 w341]
          disable-tunnel: [w335 w341] -> w329
          disable-tunnel: w328 -> [w334 _]
          frame condition #0 (active) {
            n133 = case shown="\"Busy\"" w334 {
              tunnel: w336 -> [w338 w340]
              tunnel: [w337 w339] -> w335
              frame "Idle", Default {
                n134 = call <vilib>:"Unset Busy.vi"("error in (no error)"=w338) -> ("error out"=w337:errorcluster)  [unwired: 10 in]
              }
              frame "Busy" {
                n135 = call <vilib>:"Set Busy.vi"("error in (no error)"=w340) -> ("error out"=w339:errorcluster)  [unwired: 9 in, 1 out]
              }
            }
          }
          frame condition #1 {
          }
        }
        n136 = call <vilib>:"Add State(s) to Queue__JKI_lib_State_Machine.vi"("State(s) in (\"\")"=w333) -> ("States Out"=w332:string)  [unwired: 14 in]
      }
      frame "UI: Front Panel State" {
        # "Argument"
        n137 = Unbundle By Name(w344) -> ("Core.Current VI Reference"=w343:refnum<vi>)
        n138 = case shown="\"Minimize\", \"Minimized\"" w342 {
          tunnel: w346 -> [w354 w369 w380 w393 w406]
          tunnel: [w356 w370 w382 w395 w408] -> w345
          tunnel: w343 -> [w355 w367 w381 w394 w407]
          frame "Open", "Standard", Default {
            w349 = T1."Standard" ("State")
            n139 = property class="VI"(reference=w355, error in=w354) -> (reference out=w352:refnum<vi>, error out=w353:errorcluster, "FP.State"=w351:T1)
            n140 = Not Equal?(x=w351, y=w349) -> (x != y?=w350:bool)
            n141 = case shown="True" w350 {
              tunnel: [w360 w362] -> w356
              tunnel: w353 -> [w359 w362]
              tunnel: w352 -> [w358 _]
              tunnel: w349 -> [w357 _]
              frame True {
                n142 = invoke class="VI" method="FP.Open"(reference=w358, error in=w359, "Activate"=TRUE, "State"=w357) -> (error out=w360:errorcluster)  [unwired: 1 in, 4 out]
              }
              frame False {
              }
            }
          }
          frame "Close", "Closed" {
            n143 = property class="VI"(reference=w367, error in=w369) -> (reference out=w366:refnum<vi>, error out=w368:errorcluster, "FP.State"=w364:T1)
            n144 = Not Equal?(x=w364, y=T1."Closed" ("Front Panel Window:State")) -> (x != y?=w363:bool)
            n145 = case shown="True" w363 {
              tunnel: [w371 w374] -> w370
              tunnel: w368 -> [w371 w373]
              tunnel: w366 -> [_ w372]
              frame False {
              }
              frame True {
                n146 = invoke class="VI" method="FP.Close"(reference=w372, error in=w373) -> (error out=w374:errorcluster)  [unwired: 1 in, 2 out]
              }
            }
          }
          frame "Hidden", "Hide" {
            w375 = T1."Hidden" ("State")
            n147 = property class="VI"(reference=w381, error in=w380) -> (reference out=w378:refnum<vi>, error out=w379:errorcluster, "FP.State"=w377:T1)
            n148 = Not Equal?(x=w377, y=w375) -> (x != y?=w376:bool)
            n149 = case shown="True" w376 {
              tunnel: [w386 w387] -> w382
              tunnel: w379 -> [w385 w387]
              tunnel: w378 -> [w384 _]
              tunnel: w375 -> [w383 _]
              frame True {
                n150 = invoke class="VI" method="FP.Open"(reference=w384, error in=w385, "State"=w383) -> (error out=w386:errorcluster)  [unwired: 2 in, 4 out]
              }
              frame False {
              }
            }
          }
          frame "Minimize", "Minimized" {
            w388 = T1."Minimized" ("State")
            n151 = property class="VI"(reference=w394, error in=w393) -> (reference out=w391:refnum<vi>, error out=w392:errorcluster, "FP.State"=w390:T1)
            n152 = Not Equal?(x=w390, y=w388) -> (x != y?=w389:bool)
            n153 = case shown="True" w389 {
              tunnel: [w399 w400] -> w395
              tunnel: w392 -> [w398 w400]
              tunnel: w391 -> [w397 _]
              tunnel: w388 -> [w396 _]
              frame True {
                n154 = invoke class="VI" method="FP.Open"(reference=w397, error in=w398, "State"=w396) -> (error out=w399:errorcluster)  [unwired: 2 in, 4 out]
              }
              frame False {
              }
            }
          }
          frame "Maximize", "Maximized" {
            w401 = T1."Maximized" ("State")
            n155 = property class="VI"(reference=w407, error in=w406) -> (reference out=w404:refnum<vi>, error out=w405:errorcluster, "FP.State"=w403:T1)
            n156 = Not Equal?(x=w403, y=w401) -> (x != y?=w402:bool)
            n157 = case shown="True" w402 {
              tunnel: [w412 w413] -> w408
              tunnel: w405 -> [w411 w413]
              tunnel: w404 -> [w410 _]
              tunnel: w401 -> [w409 _]
              frame True {
                n158 = invoke class="VI" method="FP.Open"(reference=w410, error in=w411, "State"=w409) -> (error out=w412:errorcluster)  [unwired: 2 in, 4 out]
              }
              frame False {
              }
            }
          }
        }
        n159 = call <vilib>:"Add State(s) to Queue__JKI_lib_State_Machine.vi"("State(s) in (\"\")"=w348) -> ("States Out"=w347:string)  [unwired: 14 in]
      }
      frame "---------- Macro ----------" {
        n160 = call <vilib>:"Add State(s) to Queue__JKI_lib_State_Machine.vi"("State(s) in (\"\")"=w417) -> ("States Out"=w416:string)  [unwired: 14 in]
      }
      frame "Macro: Initialize" {
        w418 = "Data: Initialize\nInitialize Core Data\nUI: Initialize\n//UI: Front Panel State >> Open\nAPI: Refresh Stored Scripts"  # Data: Initialize Initialize Core Data UI: Initialize //UI: Front Panel State >> Open API: Refresh Stored Scripts
        n161 = call <vilib>:"Add State(s) to Queue__JKI_lib_State_Machine.vi"("State(s) in Front (\"\")"=w418, "State(s) in (\"\")"=w422) -> ("States Out"=w421:string)  [unwired: 13 in]
      }
      frame "Macro: Exit" {
        n162 = Unbundle By Name(w430) -> ("Core.Close Panel on Exit?"=w429:bool)
        n163 = Select(t="UI: Front Panel State >> Close", s=w429, f="") -> (s? t:f=w426:string)
        n164 = call <vilib>:"Add State(s) to Queue__JKI_lib_State_Machine.vi"("State(s) in Front (\"\")"="//Exit Sub-Modules ", "State(s) in (\"\")"=w426, "State(s) at Back (\"\")"="Data: Cleanup\nExit") -> ("States Out"=w424:string)  [unwired: 12 in]
        n165 = call <vilib>:"Add State(s) to Queue__JKI_lib_State_Machine.vi"("State(s) in Front (\"\")"=w424, "State(s) in (\"\")"=w433) -> ("States Out"=w432:string)  [unwired: 13 in]
      }
      frame "---------- API ----------" {
      }
      frame "API: Run Scripts" {
        n166 = control-ref of="Scripts"() -> (w447:refnum<vi>)
        n167 = property class="LstBox (strict)"(reference=w447, "SelColor"=u32 3644238) -> (reference out=w446:refnum<vi>, "Item Names"=w439:string[])  [unwired: 1 in, 1 out]
        n168 = Array Size(array=w439) -> (size(s)=w440:i32)
        n169 = for {
          tunnel: w439 -> [w466] mode=indexing
          tunnel: [w465] -> w442
          shift-right: [w476] -> w443
          shift-left: w446 -> [w478]
          tunnel: TRUE ("Running") -> [w475]
          tunnel: [FALSE ("Running")] -> w437
          tunnel: w440 -> [w469]
          tunnel: ["Stop"] -> w438
          i -> [w472]
          stop <- w477 stop-if-true
          # "#CSM-TODO"
          n170 = local write "Running"(w475) -> ()
          n171 = Subtract(x=w472, y=5 ("upper limit")) -> (x-y=w470:i32)
          n172 = call "CSM - Run Script.vi"("CSM Scripts"=w466, "Wait (5000ms)"=100) -> ("error out"=w465:errorcluster)  [unwired: 11 in, 2 out]
          n173 = Wait (ms)(milliseconds to wait=u32 50) -> ()  [unwired: 1 out]
          n174 = In Range and Coerce(upper limit=w469, x=w470, lower limit=0) -> (coerced(x)=w473:i32)  [unwired: 1 out]
          n175 = property class="LstBox (strict)"(reference=w478, "Value"=w472, "Top Row"=w473) -> (reference out=w476:refnum<vi>)  [unwired: 1 in, 1 out]
          n176 = Or(x="Stop", y=w465) -> (x .or. y?=w477:bool)
        }
        n177 = local write "Running"(w437) -> ()
        n178 = local write "Stop"(w437) -> ()
        n179 = case shown="Error" w442 {
          tunnel: w443 -> [_ w462]
          frame No Error {
          }
          frame Error {
            n180 = property class="LstBox (strict)"(reference=w462, "SelColor"=u32 16711680) -> ()  [unwired: 1 in, 2 out]
          }
        }
        n181 = case shown="False" w438 {
          tunnel: [w454 w460] -> w445
          tunnel: w443 -> [w453 _]
          tunnel: w442 -> [w452 w460]
          frame False {
            n182 = disable-structure shown="Enabled" {
              disable-tunnel: [w457 w459] -> w454
              disable-tunnel: w453 -> [w456 _]
              disable-tunnel: w452 -> [w455 w459]
              frame Disabled {
                n183 = property class="LstBox (strict)"(reference=w456, error in=w455, "Value"=-1) -> (error out=w457:errorcluster)  [unwired: 1 out]
              }
              frame Enabled {
              }
            }
          }
          frame True {
          }
        }
        n184 = call <vilib>:"Add State(s) to Queue__JKI_lib_State_Machine.vi"("State(s) in (\"\")"=w451) -> ("States Out"=w450:string)  [unwired: 14 in]
        n185 = call <vilib>:"Simple Error Handler.vi"("error in (no error)"=w445) -> ()  [unwired: 4 in, 5 out]
      }
      frame "API: Run Scripts From Start to This Line" {
        n186 = control-ref of="Scripts"() -> (w492:refnum<vi>)
        n187 = property class="LstBox (strict)"(reference=w492, "SelColor"=u32 3644238) -> (reference out=w491:refnum<vi>, "Item Names"=w482:string[], "Value"=w480:i32)  [unwired: 1 in, 1 out]
        n188 = Increment(x=w480) -> (x+1=w479:i32)
        n189 = Array Subset(array=w482, length=w479) -> (w481:string[])  [unwired: 1 in]
        n190 = Array Size(array=w481) -> (size(s)=w485:i32)
        n191 = for {
          tunnel: w481 -> [w513] mode=indexing
          tunnel: [w512] -> w487
          shift-right: [w522] -> w488
          shift-left: w491 -> [w523]
          tunnel: TRUE ("Running") -> [w521]
          tunnel: [FALSE ("Running")] -> w483
          tunnel: w485 -> [w515]
          tunnel: [w509] -> w484
          i -> [w518]
          stop <- w510 stop-if-true
          # "#CSM-TODO"
          n192 = local write "Running"(w521) -> ()
          n193 = call "CSM - Run Script.vi"("CSM Scripts"=w513, "Wait (5000ms)"=100) -> ("error out"=w512:errorcluster)  [unwired: 11 in, 2 out]
          n194 = Subtract(x=w518, y=5 ("upper limit")) -> (x-y=w516:i32)
          n195 = In Range and Coerce(upper limit=w515, x=w516, lower limit=0) -> (coerced(x)=w519:i32)  [unwired: 1 out]
          n196 = property class="LstBox (strict)"(reference=w523, "Value"=w518, "Top Row"=w519) -> (reference out=w522:refnum<vi>)  [unwired: 1 in, 1 out]
          n197 = Wait (ms)(milliseconds to wait=u32 100) -> ()  [unwired: 1 out]
          n198 = local read "Stop"() -> (w509:bool)
          n199 = Or(x=w509, y=w512) -> (x .or. y?=w510:bool)
        }
        n200 = local write "Running"(w483) -> ()
        n201 = local write "Stop"(w483) -> ()
        n202 = case shown="Error" w487 {
          tunnel: w488 -> [_ w507]
          frame No Error {
          }
          frame Error {
            n203 = property class="LstBox (strict)"(reference=w507, "SelColor"=u32 16711680) -> ()  [unwired: 1 in, 2 out]
          }
        }
        n204 = case shown="False" w484 {
          tunnel: [w499 w505] -> w490
          tunnel: w488 -> [w498 _]
          tunnel: w487 -> [w497 w505]
          frame False {
            n205 = disable-structure shown="Enabled" {
              disable-tunnel: [w502 w504] -> w499
              disable-tunnel: w498 -> [w501 _]
              disable-tunnel: w497 -> [w500 w504]
              frame Disabled {
                n206 = property class="LstBox (strict)"(reference=w501, error in=w500, "Value"=-1) -> (error out=w502:errorcluster)  [unwired: 1 out]
              }
              frame Enabled {
              }
            }
          }
          frame True {
          }
        }
        n207 = call <vilib>:"Add State(s) to Queue__JKI_lib_State_Machine.vi"("State(s) in (\"\")"=w496) -> ("States Out"=w495:string)  [unwired: 14 in]
        n208 = call <vilib>:"Simple Error Handler.vi"("error in (no error)"=w490) -> ()  [unwired: 4 in, 5 out]
      }
      frame "API: Run Scripts From This Line to End" {
        n209 = control-ref of="Scripts"() -> (w536:refnum<vi>)
        n210 = property class="LstBox (strict)"(reference=w536, "SelColor"=u32 3644238) -> (reference out=w535:refnum<vi>, "Item Names"=w526:string[], "Value"=w524:i32)  [unwired: 1 in, 1 out]
        n211 = Array Subset(array=w526, index=w524) -> (w525:string[])  [unwired: 1 in]
        n212 = Array Size(array=w525) -> (size(s)=w529:i32)
        n213 = for {
          tunnel: w525 -> [w560] mode=indexing
          tunnel: [w559] -> w531
          shift-right: [w568] -> w532
          shift-left: w535 -> [w569]
          tunnel: TRUE ("Running") -> [w567]
          tunnel: [FALSE ("Running")] -> w527
          tunnel: w529 -> [w562]
          tunnel: [w556] -> w528
          tunnel: w524 -> [w554]
          i -> [w555]
          stop <- w557 stop-if-true
          # "#CSM-TODO"
          n214 = Add(x=w555, y=w554) -> (x+y=w553:i32)
          n215 = local write "Running"(w567) -> ()
          n216 = Subtract(x=w553, y=5 ("upper limit")) -> (x-y=w563:i32)
          n217 = In Range and Coerce(upper limit=w562, x=w563, lower limit=0) -> (coerced(x)=w565:i32)  [unwired: 1 out]
          n218 = call "CSM - Run Script.vi"("CSM Scripts"=w560, "Wait (5000ms)"=100) -> ("error out"=w559:errorcluster)  [unwired: 11 in, 2 out]
          n219 = property class="LstBox (strict)"(reference=w569, "Value"=w553, "Top Row"=w565) -> (reference out=w568:refnum<vi>)  [unwired: 1 in, 1 out]
          n220 = Wait (ms)(milliseconds to wait=u32 100) -> ()  [unwired: 1 out]
          n221 = local read "Stop"() -> (w556:bool)
          n222 = Or(x=w556, y=w559) -> (x .or. y?=w557:bool)
        }
        n223 = local write "Running"(w527) -> ()
        n224 = local write "Stop"(w527) -> ()
        n225 = case shown="Error" w531 {
          tunnel: w532 -> [_ w551]
          frame No Error {
          }
          frame Error {
            n226 = property class="LstBox (strict)"(reference=w551, "SelColor"=u32 16711680) -> ()  [unwired: 1 in, 2 out]
          }
        }
        n227 = case shown="False" w528 {
          tunnel: [w543 w549] -> w534
          tunnel: w532 -> [w542 _]
          tunnel: w531 -> [w541 w549]
          frame False {
            n228 = disable-structure shown="Enabled" {
              disable-tunnel: [w546 w548] -> w543
              disable-tunnel: w542 -> [w545 _]
              disable-tunnel: w541 -> [w544 w548]
              frame Disabled {
                n229 = property class="LstBox (strict)"(reference=w545, error in=w544, "Value"=-1) -> (error out=w546:errorcluster)  [unwired: 1 out]
              }
              frame Enabled {
              }
            }
          }
          frame True {
          }
        }
        n230 = call <vilib>:"Add State(s) to Queue__JKI_lib_State_Machine.vi"("State(s) in (\"\")"=w540) -> ("States Out"=w539:string)  [unwired: 14 in]
        n231 = call <vilib>:"Simple Error Handler.vi"("error in (no error)"=w534) -> ()  [unwired: 4 in, 5 out]
      }
      frame "API: Refresh Stored Scripts" {
        n232 = call <vilib>:"Add State(s) to Queue__jki_lib_state_machine.vi"("State(s) in Front (\"\")"="Action: Refresh Script List\nAction: Refresh Scripts" ("State(s) in Front (\"\")"), "State(s) in (\"\")"=w571) -> ("States Out"=w572:string)  [unwired: 13 in]
      }
      frame "---------------- Action --------------" {
      }
      frame "Action: Refresh Script List" {
        n233 = property on="List" class="CmbBox"() -> ("Value"=w586:string)  [unwired: 2 in, 2 out]
        n234 = call "lvcsm List Sesctions.vi"() -> ("Section Names"=w589:string[])  [unwired: 10 in, 1 out]
        n235 = for {
          tunnel: w589 -> [w598] mode=indexing
          tunnel: [w596] -> w588 mode=indexing if=w594
          shift-right: [w593] -> w585
          shift-left: w586 -> [w593]
          n236 = Match Pattern(string=w598, regular expression="^CSMScript.") -> (after substring=w596:string, offset past match=w595:i32)  [unwired: 1 in, 2 out]
          n237 = Greater Or Equal To 0?(x=w595) -> (x >= 0?=w594:bool)
        }
        n238 = Build Array (concatenate)("<default>" ("regular expression"), w588) -> (w580:string[])
        n239 = To Lower Case(string=w580) -> (all lower case string=w579:string[])
        n240 = To Lower Case(string=w585) -> (all lower case string=w578:string)
        n241 = Search 1D Array(1D array=w579, element=w578) -> (index of element=w584:i32)  [unwired: 1 in]
        n242 = Max & Min(x=w584, y=0) -> (max(x,y)=w583:i32)  [unwired: 1 out]
        n243 = Index Array(array=w580, index=w583) -> (element=w581:string)
        n244 = property on="List" class="CmbBox"("Strings[]"=w580, "Value"=w581) -> ()  [unwired: 2 in, 2 out]
      }
      frame "Action: Refresh Scripts" {
        n245 = property on="List" class="CmbBox"() -> ("Value"=w600:string)  [unwired: 2 in, 2 out]
        n246 = call "lvcsm Read Cluster.vim"("Sub-section (\"\")"=w600, "Section"="CSMScript" ("CSM Name"), "Default Prototype"=cluster{"Item":string[]} {"Item"=[]}) -> ("Cluster (Dup)"=w603:cluster{"Item":string[]})  [unwired: 7 in, 1 out]
        n247 = Unbundle By Name(w603) -> ("Item"=w599:string[])
        n248 = property on="Scripts" class="LstBox (strict)"("Item Names"=w599, "Value"=-1 ("Scripts")) -> ()  [unwired: 2 in, 2 out]
      }
      frame "Action: Save Scripts" {
        n249 = property on="List" class="CmbBox"() -> ("Value"=w611:string)  [unwired: 2 in, 2 out]
        n250 = case shown="\"\", \"<default>\"" w611 {
          selector: w611 -> [w620 _]
          tunnel: [w620 w621] -> w610
          frame Default {
          }
          frame "", "<default>" {
            n251 = call "Save as Script"() -> ("Script"=w621:string)  [unwired: 17 in, 2 out]
          }
        }
        n252 = case shown="Default" w610 {
          selector: w610 -> [_ w617]
          tunnel: [_ w614] -> w609
          tunnel: w608 -> [_ w614]
          frame "" {
          }
          frame Default {
            n253 = property on="Scripts" class="LstBox (strict)"() -> ("Item Names"=w615:string[])  [unwired: 2 in, 2 out]
            n254 = Bundle By Name(cluster=cluster{"Item":string[]} {"Item"=[]}, "Item"=w615) -> (w616:cluster{"Item":string[]})
            n255 = call "lvcsm Write Cluster.vim"("Sub-section (\"\")"=w617, "Section"="CSMScript" ("CSM Name"), "Configuration"=w616) -> ()  [unwired: 8 in, 1 out]
          }
        }
      }
      frame "Action: Delete Script" {
        n256 = property on="List" class="CmbBox"() -> ("Value"=w622:string)  [unwired: 2 in, 2 out]
        n257 = case shown="Default" w622 {
          selector: w622 -> [w627 _]
          frame Default {
            n258 = call "lvcsm Delete Section.vi"("Sub-section (\"\")"=w627, "Section"="CSMScript" ("CSM Name")) -> ()  [unwired: 9 in, 1 out]
          }
          frame "", "<default>" {
          }
        }
      }
      frame "Action: DblClick", "Action: Run Single Command" {
        n259 = call "CSM - Convert HexStr to Data.vi"("HEX String"=w632) -> ("Variant"=w634:variant, "error out"=w635:errorcluster)  [unwired: 7 in]
        n260 = Variant To Data(error in=w635, type="" ("Init State(\"Macro: Initialize\")"), Variant=w634) -> (data=w631:string, error out=w630:errorcluster)
        n261 = case shown="Default" w631 {
          selector: w631 -> [_ w651]
          tunnel: w632 -> [_ w643]
          tunnel: w630 -> [_ w647]
          tunnel: TRUE ("Running") -> [_ w646]
          tunnel: [_ FALSE ("Running")] -> w628
          frame "" {
          }
          frame Default {
            n262 = local write "Running"(w646) -> ()
            n263 = call "Remove Comments from Single-line.vi"("single-line text"=w651) -> ("single-line text without comments"=w650:string)  [unwired: 2 in]
            n264 = call "Split Single-line Message.vi"("single-line text"=w650) -> ("operator"=w649:string, "source/target"=w648:string)  [unwired: 6 in, 2 out]
            n265 = case shown="\"-@\"" w649 {
              tunnel: [_ "CSM: Message Excuted" ("State") w660] -> _
              tunnel: w648 -> [_ _ w659]
              tunnel: [_ _BroadcastDef."CSM: Message Excuted" ("Broadcast") w658] -> w639
              frame Default {
              }
              frame "-@" {
              }
              frame "->", "->|" {
                n266 = case shown="Default" w659 {
                  tunnel: ["CSM: Registration Action Excuted" ("State") "CSM: Message Excuted" ("State")] -> w660
                  tunnel: [_BroadcastDef."CSM: Registration Action Excuted" ("Broadcast") _BroadcastDef."CSM: Message Excuted" ("Broadcast")] -> w658
                  frame "register", "register as interrupt", "register as status", "unregister" {
                  }
                  frame Default {
                  }
                }
              }
            }
            n267 = call "CSM - Run Script.vi"("CSM Scripts"=w651, "Wait (5000ms)"=100, "error in (no error)"=w647) -> ("error out"=w640:errorcluster)  [unwired: 10 in, 2 out]
            n268 = Wait (ms)(milliseconds to wait=u32 100) -> ()  [unwired: 1 out]
            n269 = call "_Broadcast Message.vi"("Argument(\"\")"=w643, "Broadcast"=w639) -> ()  [unwired: 9 in, 1 out]
            n270 = control-ref of="Scripts"() -> (w641:refnum<vi>)
            n271 = case shown="No Error" w640 {
              tunnel: w641 -> [w653 w655]
              frame No Error {
                n272 = property class="LstBox (strict)"(reference=w653, "SelColor"=u32 3644238) -> ()  [unwired: 1 in, 2 out]
              }
              frame Error {
                n273 = property class="LstBox (strict)"(reference=w655, "SelColor"=u32 16711680) -> ()  [unwired: 1 in, 2 out]
              }
            }
            n274 = call <vilib>:"Simple Error Handler.vi"("error in (no error)"=w640) -> ()  [unwired: 4 in, 5 out]
          }
        }
        n275 = local write "Running"(w628) -> ()
      }
    }
  }
